vi "Shutdown.vi"(8 "error in (no error)":errorcluster, 11 "VISA Client in":refnum<class "Serial Client.lvclass">) -> (0 "error out":errorcluster, 3 "VISA Client out":refnum<class "Serial Client.lvclass">)   [LabVIEW 2020, in "Stream-Serial.lvlib" / "Serial Client.lvclass"]
uses:
  Serial Client.lvclass
  C:/Program Files (x86)/National Instruments/LabVIEW 2020/vi.lib/IlluminatedG/lv-stream/Connection/Connection.lvclass
  Client Command.ctl
  <vilib>/IlluminatedG/lv-stream/Connection/State.ctl
  Serial Client.lvclass/Serial Client.ctl
  Stream-Serial.lvlib
  <vilib>/IlluminatedG/lv-stream/Connection/Connection.lvclass
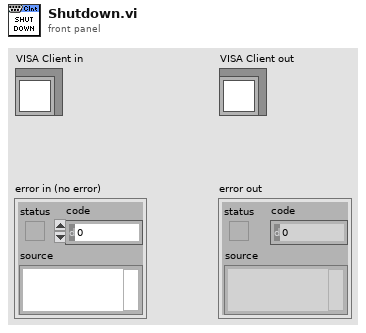
[diagram p1: front panel]
types:
  T1 = typedef "Stream.lvlib/Connection.lvclass/State.ctl" = enum16{"Closed", "Idle", "Connecting", "Connected", "Shutdown"}
  T2 = typedef "Stream-Serial.lvlib/Client Command.ctl" = enum16{"Connect", "Close", "Shutdown", "Reconnect"}
  T3 = typedef "Stream-Serial.lvlib/Command Queue.ctl" = refnum<queue>
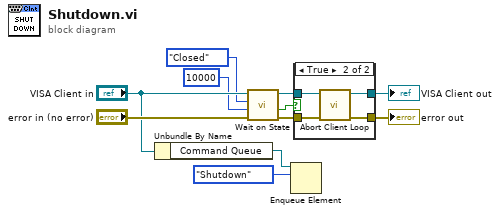
[diagram p0: block diagram]
diagram:
  n1 = Unbundle By Name("VISA Client in") -> ("Command Queue"=w9:T3)
  n2 = call <vilib>:"Wait on State.vi"("error in (no error)"="error in (no error)", "Timeout ms (-1)"=10000, "State"=State."Closed", "Connection in"="VISA Client in") -> ("error out"=w4:errorcluster, "Timed Out?"=w3:bool, "Connection out"=w5:refnum<class "Serial Client.lvclass">)  [unwired: 5 in]
  n3 = Enqueue Element(queue=w9, element=Client_Command."Shutdown") -> ()  [unwired: 2 in, 3 out]
  n4 = case shown="True" w3 {
    tunnel: w5 -> [w12 w16]
    tunnel: w4 -> [w13 w17]
    tunnel: [w12 w15] -> w2
    tunnel: [w13 w14] -> w1
    frame False {
    }
    frame True {
      n5 = call "Abort Client Loop.vi"("error in (no error)"=w17, "VISA Client in"=w16) -> ("error out"=w14:errorcluster, "VISA Client out"=w15:refnum<class "Serial Client.lvclass">)  [unwired: 8 in]
    }
  }
  "error out" <- w1
  "VISA Client out" <- w2
